vi "getObjValue.vi"(8 "error in (no error)":errorcluster, 10 "NumberOfAcitveVariables":dbl, 11 "OptimizationSimulation in":refnum<class "OptimizationSimulation.lvclass">) -> (0 "error out":errorcluster, 3 "result":dbl)   [LabVIEW 2020, in "OptimizationSimulation.lvclass"]
uses:
  OptimizationSimulation.lvclass
  OptimizationSimulation.lvclass/OptimizationSimulation.ctl
  ExpressFormulaBlockNode.xnode
  NI_AALBase.lvlib
panel:
  out "Result":dbl
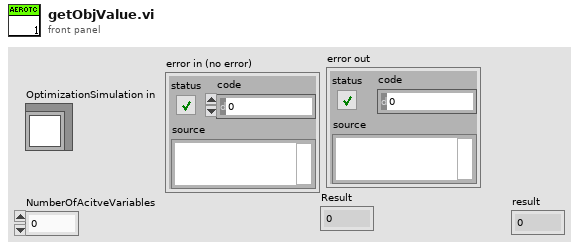
[diagram p1: front panel]
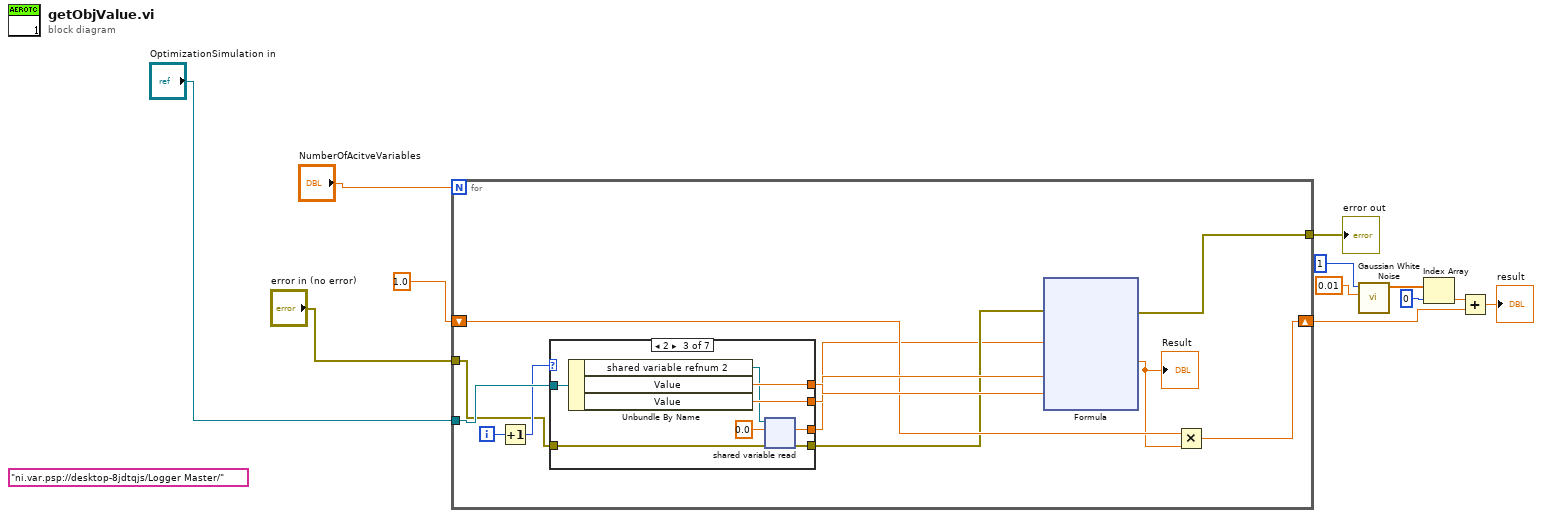
[diagram p0: block diagram]
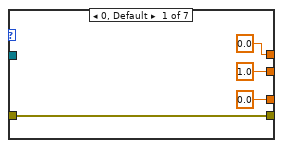
[diagram p2: hidden frame]
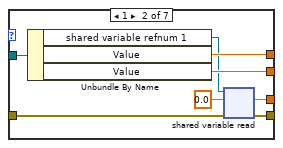
[diagram p3: hidden frame]
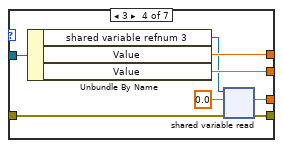
[diagram p4: hidden frame]
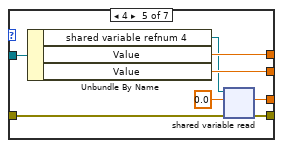
[diagram p5: hidden frame]
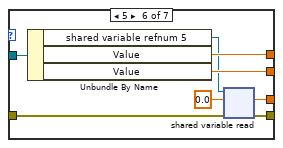
[diagram p6: hidden frame]
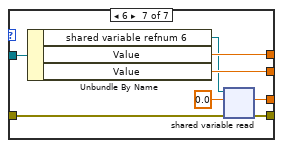
[diagram p7: hidden frame]
diagram:
  (unwired) "ni.var.psp://desktop-8jdtqjs/Logger Master/"
  n1 = for {
    N: "NumberOfAcitveVariables" -> [_]
    tunnel: "OptimizationSimulation in" -> [w24]
    tunnel: "error in (no error)" -> [w15]
    tunnel: [w19] -> w10
    shift-right: [w16] -> w6
    shift-left: 1.0 ("Result") -> [w18]
    i -> [w23]
    n2 = Increment(x=w23) -> (x+1=w22:i32)
    n3 = case shown="2" w22 {
      tunnel: w24 -> [_ w48 w56 w64 w72 w80 w88]
      tunnel: [0.0 ("Value") w47 w54 w62 w70 w78 w86] -> w21
      tunnel: [1.0 ("Value") w46 w55 w63 w71 w79 w87] -> w20
      tunnel: w15 -> [w38 w43 w53 w61 w69 w77 w85]
      tunnel: [w38 w42 w52 w60 w68 w76 w84] -> w14
      tunnel: [0.0 w41 w49 w57 w65 w73 w81] -> w13
      frame 0, Default {
      }
      frame 1 {
        n4 = Unbundle By Name(w48) -> ("shared variable refnum 1"=w44:refnum<k21>, "Value"=w47:dbl, "Value"=w46:dbl)
        n5 = shared-variable-read(w44, w43, 0.0) -> (w42:errorcluster, w41:dbl)  [unwired: 2 out]
      }
      frame 2 {
        n6 = Unbundle By Name(w56) -> ("shared variable refnum 2"=w50:refnum<k21>, "Value"=w54:dbl, "Value"=w55:dbl)
        n7 = shared-variable-read(w50, w53, 0.0) -> (w52:errorcluster, w49:dbl)  [unwired: 2 out]
      }
      frame 3 {
        n8 = Unbundle By Name(w64) -> ("shared variable refnum 3"=w58:refnum<k21>, "Value"=w62:dbl, "Value"=w63:dbl)
        n9 = shared-variable-read(w58, w61, 0.0) -> (w60:errorcluster, w57:dbl)  [unwired: 2 out]
      }
      frame 4 {
        n10 = Unbundle By Name(w72) -> ("shared variable refnum 4"=w66:refnum<k21>, "Value"=w70:dbl, "Value"=w71:dbl)
        n11 = shared-variable-read(w66, w69, 0.0) -> (w68:errorcluster, w65:dbl)  [unwired: 2 out]
      }
      frame 5 {
        n12 = Unbundle By Name(w80) -> ("shared variable refnum 5"=w74:refnum<k21>, "Value"=w78:dbl, "Value"=w79:dbl)
        n13 = shared-variable-read(w74, w77, 0.0) -> (w76:errorcluster, w73:dbl)  [unwired: 2 out]
      }
      frame 6 {
        n14 = Unbundle By Name(w88) -> ("shared variable refnum 6"=w82:refnum<k21>, "Value"=w86:dbl, "Value"=w87:dbl)
        n15 = shared-variable-read(w82, w85, 0.0) -> (w84:errorcluster, w81:dbl)  [unwired: 2 out]
      }
    }
    n16 = xnode "Formula"("variableValue"=w13, "sigma"=w20, "mu"=w21, "error in (no error)"=w14) -> ("Result"=w17:dbl, "error out"=w19:errorcluster)
    "Result" <- w17
    n17 = Multiply(x=w18, y=w17) -> (x*y=w16:dbl)
  }
  "error out" <- w10
  n18 = call "Gaussian White Noise.vi"("standard deviation"=0.01, "samples"=1) -> ("Gaussian noise pattern"=w5:dbl[])  [unwired: 8 in, 1 out]
  n19 = Index Array(array=w5, index=0) -> (element=w3:dbl)
  n20 = Add(x=w3, y=w6) -> (x+y=→"result":dbl)
